vi "Start Single Input UI.vi"(8 "error in (no error)":errorcluster, 9 "Control Name":string, 10 "UI Stop Event":refnum<event-registration>, 11 "SubPanel in":refnum<vi>) -> (0 "error out":errorcluster, 2 "VI Reference out":refnum<vi>, 3 "SubPanel out":refnum<vi>)   [LabVIEW 2015, in "CallVIStep.lvclass"]
uses:
  CallVIStep.lvclass
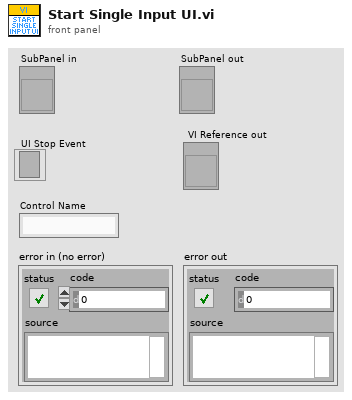
[diagram p1: front panel]
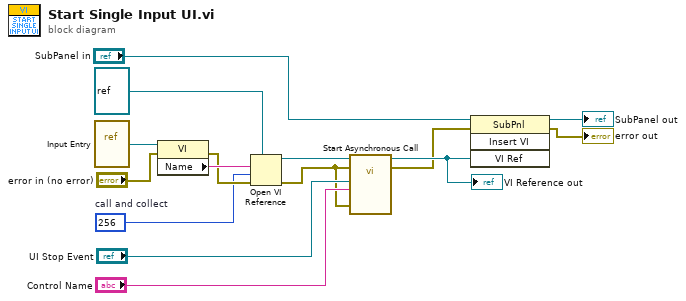
[diagram p0: block diagram]
diagram:
  w9 = 256  # call and collect
  n1 = vi-ref "Input Entry.vi"() -> (w14:refnum<vi>)
  n2 = property class="VI"(reference=w14, error in="error in (no error)") -> (error out=w10:errorcluster, "Name"=w11:string)  [unwired: 1 out]
  n3 = Open VI Reference(type specifier VI Refnum (for type only)=refnum<vi> refnum, vi path=w11, options=w9, error in (no error)=w10) -> (vi reference=w8:refnum<vi>, error out=w2:errorcluster)  [unwired: 2 in]
  n4 = call-by-ref "Start Asynchronous Call"(reference=w8, error in=w2, 8:"error in (no error)"=w2, "Control"="Control Name", "Event Registration Refnum"="UI Stop Event") -> (reference out=w15:refnum<vi>, error out=w6:errorcluster)  [unwired: 8 in, 1 out]
  "VI Reference out" <- w15
  n5 = invoke class="SubPnl" method="Insert VI"(reference="SubPanel in", error in=w6, "VI Ref"=w15) -> (reference out=→"SubPanel out":refnum<vi>, error out=→"error out":errorcluster)  [unwired: 1 in, 2 out]
